vi "get crate maps.vi"(0 "VISA in":refnum<visa-resource-name>, 11 "error in":errorcluster) -> (4 "VISA out":refnum<visa-resource-name>, 10 "Total Channel Count":i32, 15 "error out":errorcluster)   [LabVIEW 2018]
uses:
  CAEN globals.vi
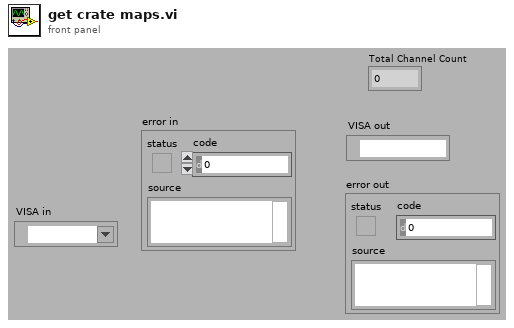
[diagram p1: front panel]
types:
  T1 = typedef "crate.ctl" = cluster{"CAENet Address":i32, "Crate Model":string, "Firmware Version":string, "Crate Map":T2[], "Total Channels":i32}
  T2 = typedef "card.ctl" = cluster{"Slot Number":i32, "Card Model":string, "Num Channels":i32, "Polarity":string, "Vmax":dbl, "Imax":dbl, "Revision":string}
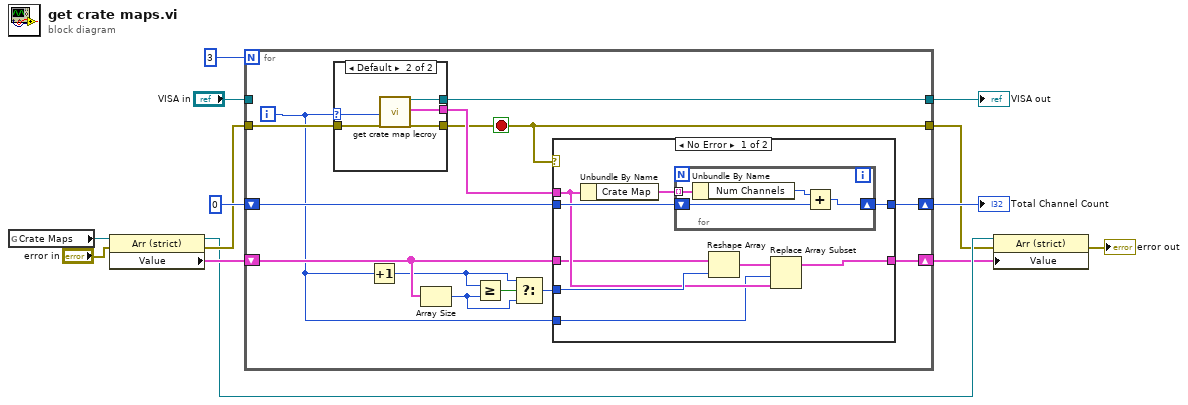
[diagram p0: block diagram]
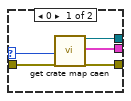
[diagram p2: hidden frame]
diagram:
  n1 = global read "CAEN globals.vi" "Crate Maps"() -> (w8:refnum<vi>)
  n2 = property class="Arr (strict)"(reference=w8, error in="error in") -> (reference out=w4:refnum<vi>, error out=w6:errorcluster, "Value"=w7:T1[])
  n3 = for {
    N: 3 ("Num crates") -> [_]
    tunnel: w6 -> [w26]
    tunnel: [w16] -> w1
    tunnel: [w25] -> w13
    tunnel: "VISA in" -> [_]
    shift-right: [w23] -> w9
    shift-left: 0 -> [w24]
    shift-right: [w17] -> w3
    shift-left: w7 -> [w18]
    i -> [w14]
    stop <- w16 stop-if-true
    n4 = case shown="Default" w14 {
      selector: w14 -> [w27 w32]
      tunnel: w26 -> [w31 w36]
      tunnel: [w30 w35] -> w25
      tunnel: [w29 w34] -> w19
      tunnel: [w28 w33] -> w16
      frame 0 {
        n5 = call "get crate map caen.vi"("Crate"=w27, "error in"=w31) -> ("VISA out"=w30:refnum<visa-resource-name>, "Crate Details"=w29:T1, "error out"=w28:errorcluster)  [unwired: 14 in, 1 out]
      }
      frame Default {
        n6 = call "get crate map lecroy.vi"("Crate"=w32, "error in"=w36) -> ("VISA out"=w35:refnum<visa-resource-name>, "Crate Details"=w34:T1, "error out"=w33:errorcluster)  [unwired: 15 in]
      }
    }
    n7 = Increment(x=w14) -> (x+1=w15:i32)
    n8 = Array Size(array=w18) -> (size(s)=w21:i32)
    n9 = Greater Or Equal?(x=w15, y=w21) -> (x >= y?=w22:bool)
    n10 = Select(t=w15, s=w22, f=w21) -> (s? t:f=w20:i32)
    n11 = case shown="No Error" w16 {
      tunnel: w24 -> [w44 w51]
      tunnel: [w43 w51] -> w23
      tunnel: w20 -> [w42 _]
      tunnel: w19 -> [w41 _]
      tunnel: w18 -> [w40 w50]
      tunnel: [w39 w50] -> w17
      tunnel: w14 -> [w38 _]
      frame No Error {
        n12 = Unbundle By Name(w41) -> ("Crate Map"=w45:T2[])
        n13 = for {
          tunnel: w45 -> [w49] mode=indexing
          shift-right: [w48] -> w43
          shift-left: w44 -> [w46]
          n14 = Unbundle By Name(w49) -> ("Num Channels"=w47:i32)
          n15 = Add(x=w47, y=w46) -> (x+y=w48:i32)
        }
        n16 = Reshape Array(w40, w42) -> (w37:T1[])
        n17 = Replace Array Subset(array=w37, new element=w41, index=w38) -> (w39:T1[])
      }
      frame Error {
      }
    }
  }
  "VISA out" <- w13
  "Total Channel Count" <- w9
  n18 = property class="Arr (strict)"(reference=w4, error in=w1, "Value"=w3) -> (error out=→"error out":errorcluster)  [unwired: 1 out]
